vi "Keyence.Main-Tune.vi"(7 "Idx":i32, 8 "error in":errorcluster, 10 "Bank":u8) -> (0 "error out":errorcluster, 1 "Tuned":bool, 2 "Code":T3, 3 "Final status":T1={"State"=enum."Init", "Ref"=refnum, "Bank"=0, "Version"="", "Model"="", "EndTS"=timestamp(0 s since 1904-01-01), "ImgPath"=path "", "Tuned"=FALSE})   [LabVIEW 2015]
uses:
  LowLevel/Keyence.CodeDetails.ctl
  Keyence.Data.Status.ctl
  Keyence.Data.Status.State.ctl
  Keyence.Action.ctl
  tools/EventLog/EventLog.EventSource.ctl
  tools/Translator/Translator.Message.ctl
  tools/EventLog/EventLog.CreateError(array).vi
  tools/Translator/Translator.Translate.Status (NoError).vi
  tools/Translator/Translator.FormatMessage.vi
  tools/EventLog/EventLog.New(array).vi
  tools/Translator/Translator.Global.vi
  tools/ErrorHandling/ErrorHandling.Create.vi
  LowLevel/Keyence.Global.vi
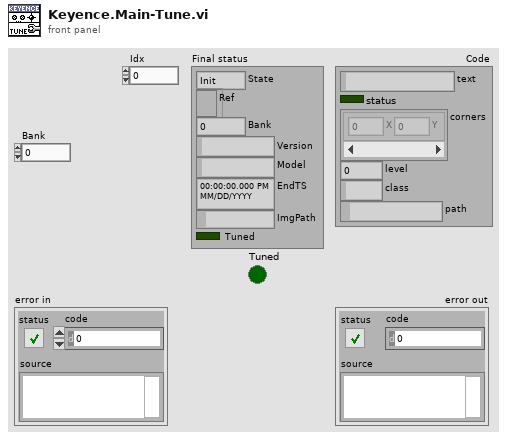
[diagram p1: front panel]
types:
  T1 = typedef "Keyence.Data.Status.ctl" = cluster{"State":T2, "Ref":refnum<k5>, "Bank":u8, "Version":string, "Model":string, "EndTS":timestamp, "ImgPath":path, "Tuned":bool}
  T2 = typedef "Keyence.Data.Status.State.ctl" = enum16{"First", "Init", "Reset", "Idle", "Scan", "Tune"}
  T3 = typedef "Keyence.CodeDetails.ctl" = cluster{"text":string, "status":bool, "corners":cluster{"X":i32, "Y":i32}[], "level":u8, "class":string, "path":path}
  T4 = typedef "Keyence.Action.ctl" = enum32{"idle", "constructor", "destructor", "--- Keyence ---", "Init", "Scan", "Tune"}
  T5 = typedef "Translator.Message.ctl" = enum16{"-", "Event confirmed", "Log out", "Log in", "Shutdown", "Cancel", "Start", "Begin time", "End time", "Duration", "Service Mode", "Ignore Results", "On", "Off", "OK", "NOK", "NOK %s", "Home", "Work", "Close", "Open", "In progress...", "Missing", "Empty", "Hardware failure", "Initial", "Out of range", "Error %d >> %s", "Error %d >> %s >> %s", "Msg %d >> %s", "Laser msg %d %s", "Laser cmd error %s %d", "Laser cmd failed %s", "Laser cmd warning %s", "Laser disconnected", "Laser status %s", "Laser already started", "Laser job unkonwn %s", "Laser job missing %s", "Laser job select failure %s", "Unable to start laser printing (%s)", "Unable to stop laser printing (%s)", "Laser marking aborted", "Unable to reset Laser Interlock (%s)", "Unable to trigger Laser. Laser not ready (%s)", "Laser job '%s' coordinates not configured", "Starting %s", "Quitting %s", "Configured", "Initializing", "Quitting", "Loading", "Running", "Stopped", "Summary", "Laser", "Do you want to continue?", "Press confirm button", "Station is not based. Do you want to exit?", "Station requires changeover. Do you want to run the test?", "Test options are not set as default. Do you want to continue?", "Product not detected. Do you want to continue?", "Product scan failed. Do you want to continue?", "Calibration", "Log out?", "System", "All", "IDLE", "Translating...%s", "Not found", "Alarm %s", "Run", "Skip", "Abort", "Repeat", "Please wait...", "Database disconnected", "Database disconnected - changeover disabled!", "Login to database successful", "Login to database failed: %d; %s", "Unable to check the product status of reference %d - database disconnected", "Unable to set the product status of reference %d - database disconnected", "Variant file backup %s", "Read steps (%s)", "Result", "Station armed!", "Station requires changeover!", "Select reference number...", "EMERGENCY BUTTON - press Control button", "EMERGENCY DOOR - press Control button", "Resetting Emergency...", "Unable to reset safety circuit - Emergency Button pressed", "Unable to reset safety circuit - Emergency Side Door open", "Station not based", "Station based", "Station not empty", "Station basing...", "No order", "Press Start to begin new order", "Scanning new order", "Order NOK. Correct or scan again", "Order OK. Press Accept", "Order ready", "Revolver incorrect", "Fork incorrect", "Revolver missing", "Revolver empty", "Container missing", "Offline results", "Door open", "Close the front door", "Press start button", "Done. Open the front door", "Error. Press Confirm button", "Remove product", "Confirm failure", "Running...", "Running...%.1f %%", "Pause", "Pause. NOK container missing", "Pause. OK container missing", "Pause. Revolver empty", "Pause. Revolver missing", "Pause. Revolver incorrect", "Pause. Fork missing", "Pause. Fork incorrect", "Pause. Too many failures", "Pause. Unable to unload", "Pause. One slot is not working", "Pause. Unable to move product to slot", "Pause. Unable to move back product pusher", "Pause. Unable to lift product", "Pause. Unable to move back product lifter", "Pause. Unable to move product arm to Work", "Pause. Unable to move product arm to NOK", "Pause. Unable to move product arm to OK", "Pause. Unable to unsuck the NOK product", "Pause. Unable to drop the NOK product", "Pause. Product OK missing", "Pause. Unable to unsuck the OK product", "Pause. Unable to drop the OK product", "Pause. ", "Stopping...", "Finalizing...", "Sequence folder '%s' is missing", "File '%s' is missing", "File '%s' is broken", "File '%s' is running", "Log file started (%s)", "Log file ended (%s)", "Log file ignored (%s)", "Log file exported (%s)", "Log file export failed (%s)", "Wrong serial number in log file", "Wrong reference number in log file", "Test steps are missing", "%s = %.3f", "Process param '%s' not found in DB", "Process param '%s' wrong order", "Process param '%s' value %.3f out of limits (%.3f; %.3f)", "Step%d param '%s' not found in DB", "Step%d param '%s' wrong order", "Step%d param '%s' value %.3f out of limits (%.3f; %.3f)", "Step%d EV '%s' not found in DB", "Step%d EV '%s' wrong order", "\"%s\" not found in DB", "\"%s\" wrong order", "\"%s\" value %.3f out of limits (%.3f; %.3f)", "\"%s\" not found in software", "Process init (%s)", "Process started", "Process restarted", "Process run", "Process done", "Process aborted", "Process aborted at work", "Process aborted at home", "Process error", "Process error at home", "Process error at work", "Process close", "Select plate from the order to process", "Do you want to start the process?", "Do you want to repeat the process?", "There is unfinished order. Do you want to put the new order?", "Product %s %d OK", "Product %s %d NOK", "Unable to unload the slot %s. Product missing in the slot", "Unable to unload the slot %s. Product already in the arm", "Unable to accept the product as OK. Product missing in slot %s", "Unable to accept the product as OK. Product could not drop into the container at slot %s", "Unable to accept the product as NOK. Product could not drop into the container at slot %s", "Scan failed. Error %s", "Scan failed. Scanner disconnected", "Scan failed. Wrong Wabco number %d, limit (%d,%d)", "Scan failed. Wrong serial number %d, limit (%d,%d)", "Scan failed. Wrong date %d, limit (%d,%d)", "Scan failed. Wrong product wabco number %d (expected %d)", "Scan failed. Wrong product serial number %d (expected > 0)", "Scan OK %s", "Scan failed. Unable to determine table position (%s)", "Scan failed. Timeout", "Tune failed. Scanner disconnected", "Tune failed. Timeout", "%s = %d", "%s = %d->%d", "Unable to set %s = %.2f - Air Pressure Inside off", "Unable to set digital output '%s' = %d", "Unable to activate air pressure inside - timeout", "Unable to activate air pressure inside - aborted", "Unable to switch on Air Main Valve - Air Pressure Inlet off", "Unable to switch on Air Main Valve - Door open", "Unable to switch off Air Main Valve - timeout", "Unable to switch off Air Main Valve - aborted", "Unable to rotate Table - timeout", "Unable to rotate Table - aborted", "Unable to rotate Table - Product Move not in Home position", "Unable to rotate Table - Air Pressure Inside off", "Unable to rotate Table - Product Lift A not in Home position", "Unable to rotate Table - Product Lift B not in Home position", "Unable to rotate Table - unlock before movement timeout", "Unable to rotate Table - lock after movement timeout", "Unable to move Table Lock to %s position - timeout", "Unable to move Table Lock to %s position - aborted", "Unable to move Table Lock to %s position - Air Pressure Inside off", "Unable to move Table Lock to %s position - Table not in position", "Unable to move Product Lift A to %s position - timeout", "Unable to move Product Lift B to %s position - timeout", "Unable to move Product Lift A to %s position - aborted", "Unable to move Product Lift B to %s position - aborted", "Unable to move Product Lift A to %s position - Air Pressure Inside off", "Unable to move Product Lift B to %s position - Air Pressure Inside off", "Unable to move Product Lift A to %s position - Table not locked", "Unable to move Product Lift B to %s position - Table not locked", "Unable to move Product Lift A to %s position - Product Arm not in Work position", "Unable to move Product Lift B to %s position - Product Arm not in Work position", "Unable to set Product Suction Gripper %s to %s - timeout", "Unable to set Product Suction Gripper %s to %s - aborted", "Unable to set Product Suction Gripper %s to %s - Air Pressure Inside off", "Unable to set Product Suction Gripper %s to %s - Table slot unkown", "Unable to move Product Arm to %s position - timeout", "Unable to move Product Arm to %s position - aborted", "Unable to move Product Arm to %s position - Air Pressure Inside off", "Unable to move Product Arm to %s position - Product Lift A not in Home position", "Unable to move Product Arm to %s position - Product Lift B not in Home position", "Unable to move Product to %s position - timeout", "Unable to move Product to %s position - aborted", "Unable to move Product to %s position - Air Pressure Inside off", "Unable to move Product to %s position - Table not in position"}
  T6 = typedef "EventLog.EventSource.ctl" = enum16{"All", "Gui", "Ref", "File", "Seq", "CPX", "Proda", "Laser", "Scan.P", "Scan.O"}
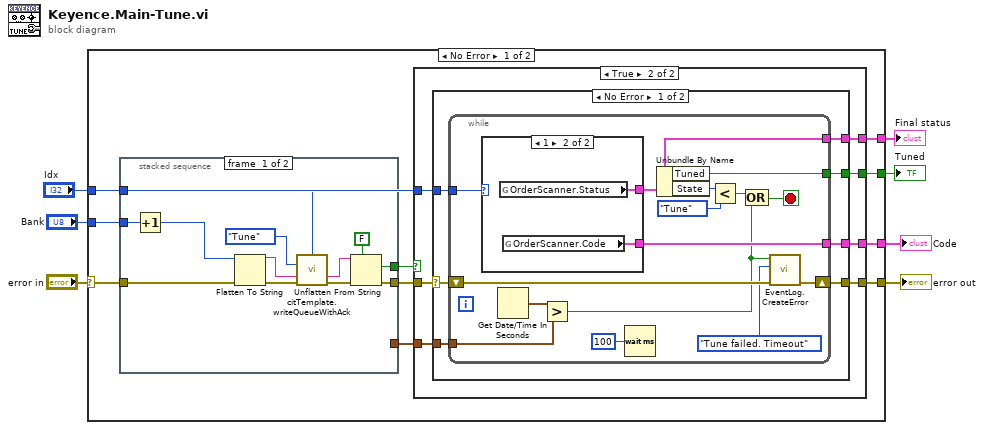
[diagram p0: block diagram]
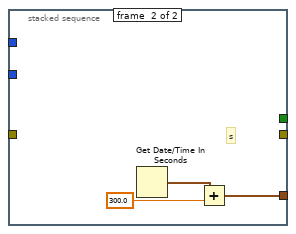
[diagram p2: hidden frame]
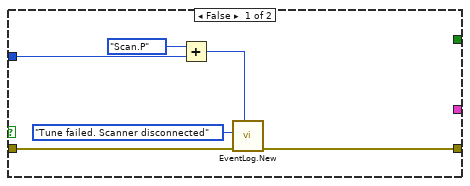
[diagram p3: hidden frame]
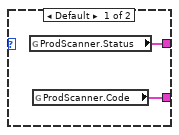
[diagram p4: hidden frame]
diagram:
  n1 = case shown="No Error" "error in" {
    selector: "error in" -> [w17 w73]
    tunnel: [w16 w73] -> w6
    tunnel: "Bank" -> [w12 _]
    tunnel: [w15 _] -> w4
    tunnel: "Idx" -> [w11 _]
    tunnel: [w9 _] -> w2
    tunnel: [w8 _] -> w1
    frame No Error {
      n2 = stacked-sequence {
        tunnel: w17 -> [w29 _]
        tunnel: w11 -> [w25 _]
        tunnel: [w21 _] -> w14
        tunnel: [w20 _] -> w13
        tunnel: w12 -> [w19 _]
        tunnel: [_ w30] -> w10
        frame #0 {
          n3 = Increment(x=w19) -> (x+1=w18:u8)
          n4 = Flatten To String(anything=w18, error in (no error)=w29) -> (data string=w27:string, error out=w28:errorcluster)  [unwired: 2 in, 1 out]
          n5 = call "citTemplate.writeQueueWithAck.vi"("instance (0)"=w25, "event in"=Keyence.Action."Tune" ("Action"), "(flatten) data in"=w27, "error in (no error)"=w28) -> ("notification data"=w23:string, "error out"=w24:errorcluster)  [unwired: 9 in, 1 out]
          n6 = Unflatten From String(type=FALSE, binary string=w23, error in (no error)=w24) -> (value=w20:bool, error out=w21:errorcluster)  [unwired: 2 in, 1 out]
        }
        frame #1 {
          # "s"
          n7 = Get Date/Time In Seconds() -> (seconds since 1Jan1904=w32:timestamp)
          n8 = Add(x=w32, y=300.0) -> (x+y=w30:timestamp)
        }
      }
      n9 = case shown="True" w13 {
        tunnel: w14 -> [w37 w45]
        tunnel: [w36 w44] -> w16
        tunnel: [_ w43] -> w15
        tunnel: w11 -> [w35 w42]
        tunnel: w10 -> [_ w41]
        tunnel: [_ w40] -> w9
        tunnel: [_ w39] -> w8
        frame False {
          n10 = Add(x=EventLog.EventSource."Scan.P" ("Source (All)"), y=w35) -> (x+y=w33:i32)
          n11 = call-poly "EventLog.New.vi"("Source (All)"=w33, "error in (no error)"=w37, "Message (-)"=Translator.Message."Tune failed. Scanner disconnected") -> ("error out"=w36:errorcluster)  [unwired: 7 in, 1 out]
        }
        frame True {
          n12 = case shown="No Error" w45 {
            selector: w45 -> [w51 w72]
            tunnel: [w50 w72] -> w44
            tunnel: [w52 _] -> w43
            tunnel: w42 -> [w49 _]
            tunnel: w41 -> [w48 _]
            tunnel: [w47 _] -> w40
            tunnel: [w46 _] -> w39
            frame No Error {
              n13 = while {
                tunnel: [w63] -> w52
                shift-right: [w57] -> w50
                shift-left: w51 -> [w62]
                tunnel: w49 -> [w61]
                tunnel: w48 -> [w60]
                tunnel: [w54] -> w47
                tunnel: [w53] -> w46
                stop <- w58 stop-if-true
                n14 = case shown="1" w61 {
                  tunnel: [w69 w71] -> w54
                  tunnel: [w68 w70] -> w63
                  frame Default {
                    n15 = global read "Keyence.Global.vi" "ProdScanner.Status"() -> (w69:T1)
                    n16 = global read "Keyence.Global.vi" "ProdScanner.Code"() -> (w68:T3)
                  }
                  frame 1 {
                    n17 = global read "Keyence.Global.vi" "OrderScanner.Status"() -> (w71:T1)
                    n18 = global read "Keyence.Global.vi" "OrderScanner.Code"() -> (w70:T3)
                  }
                }
                n19 = Get Date/Time In Seconds() -> (seconds since 1Jan1904=w59:timestamp)
                n20 = Greater?(x=w59, y=w60) -> (0:w56:bool)
                n21 = Wait (ms)(milliseconds to wait=u32 100) -> ()  [unwired: 1 out]
                n22 = Unbundle By Name(w54) -> ("Tuned"=w53:bool, "State"=w67:T2)
                n23 = Less?(x=w67, y=Keyence.Data.Status.State."Tune") -> (x < y?=w65:bool)
                n24 = Compound Arithmetic op=OR(w65, w56) -> (w58:bool)
                n25 = call-poly "EventLog.CreateError.vi"("error in"=w62, "msg"=Translator.Message."Tune failed. Timeout", "create (T)"=w56) -> ("error out"=w57:errorcluster)  [unwired: 7 in, 1 out]
              }
            }
            frame Error {
            }
          }
        }
      }
    }
    frame Error {
    }
  }
  "error out" <- w6
  "Code" <- w4
  "Final status" <- w2
  "Tuned" <- w1
